vi "Texto Pasante.vi"() -> ()   [LabVIEW 2010]
panel:
  in  "Dejar espacio":bool
  in  "Columnas":u32=30
  out "Array booleano":bool[][](array[boolean])
  in  "Velocidad [columnas / segundo]":dbl(slide)=21.09090909090909 scale=1.0..40.0
  in  "Texto":string
  in  "Abrir fuente":bool
  in  "Salir":bool
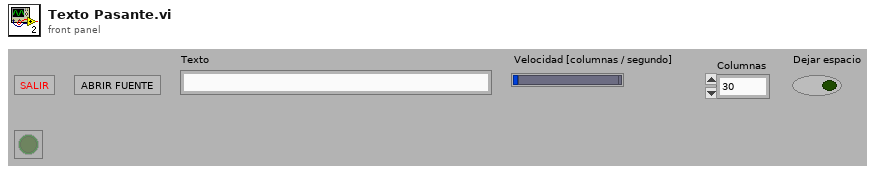
[diagram p1: front panel]
types:
  T1 = enum16{"open", "replace", "create", "open or create", "replace or create", "replace or create with confirmation"}
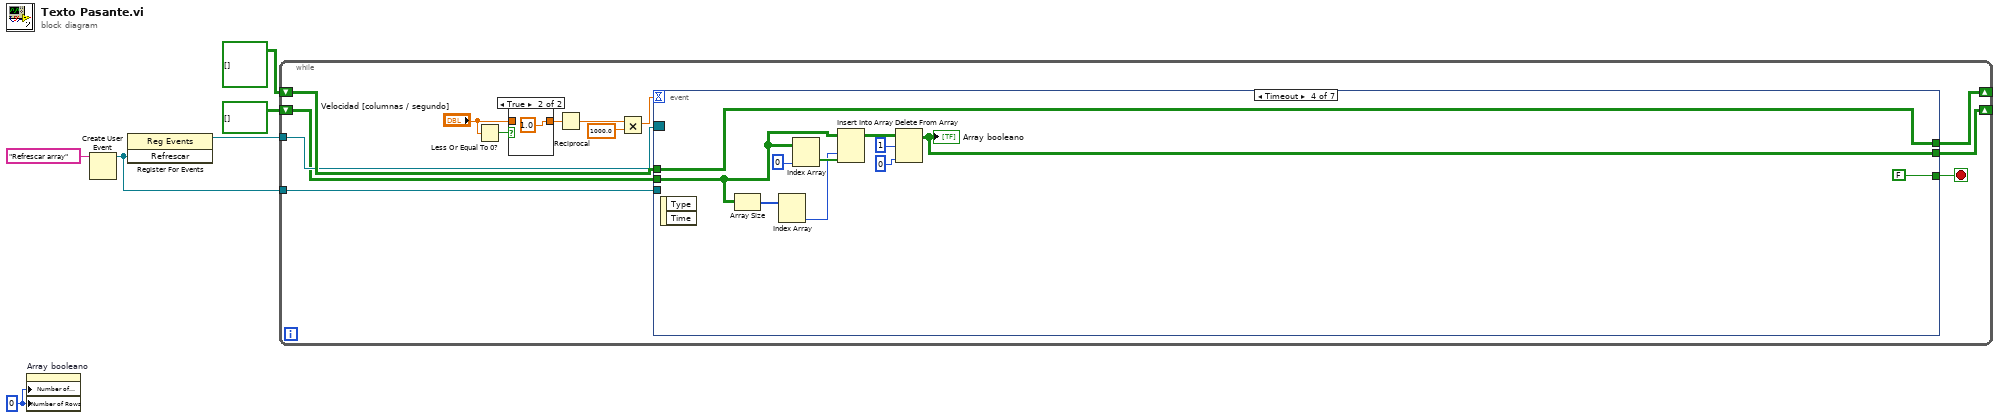
[diagram p0: block diagram]
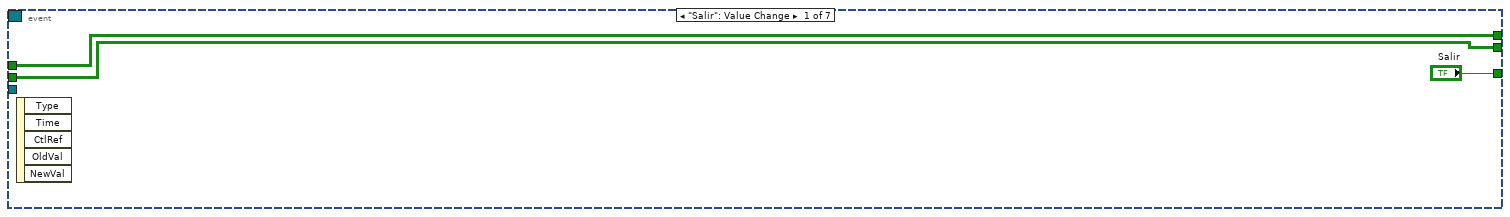
[diagram p3: hidden frame]
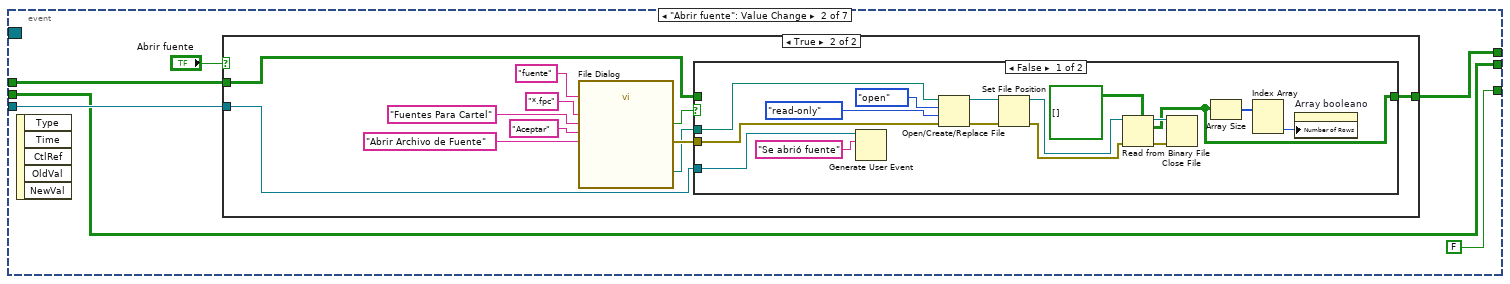
[diagram p4: hidden frame]
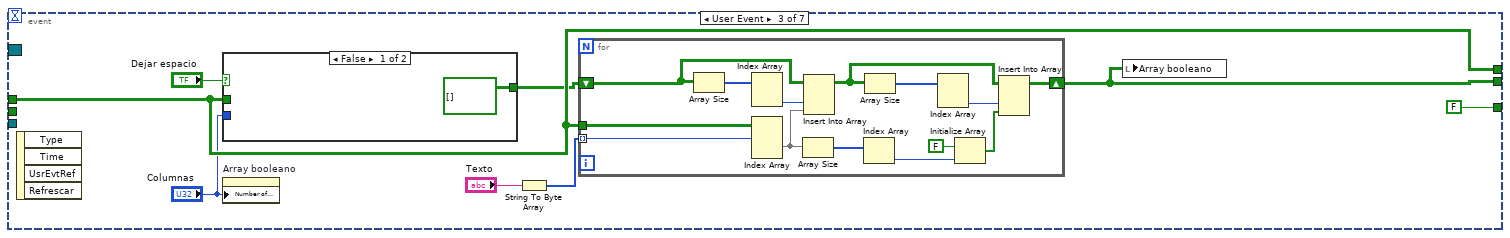
[diagram p7: hidden frame]
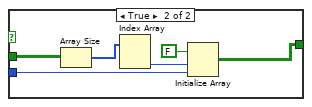
[diagram p8: hidden frame]
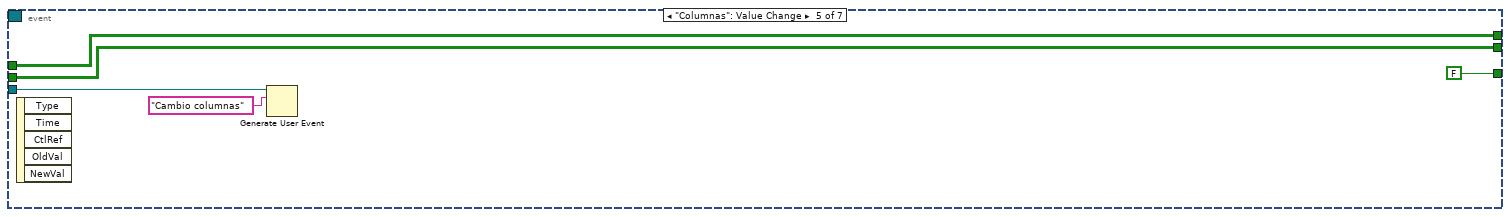
[diagram p9: hidden frame]
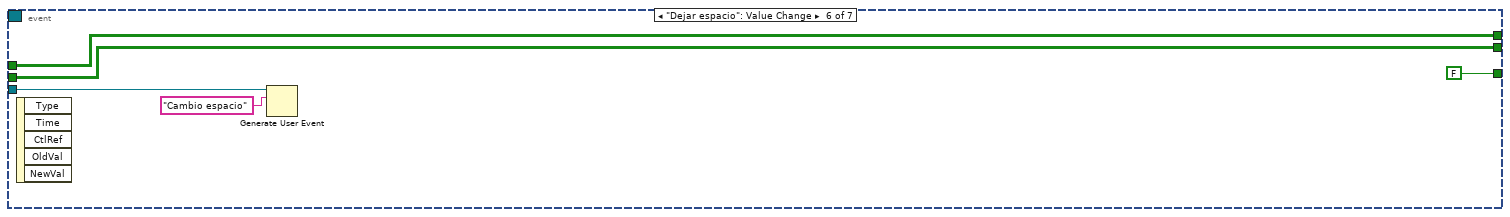
[diagram p10: hidden frame]
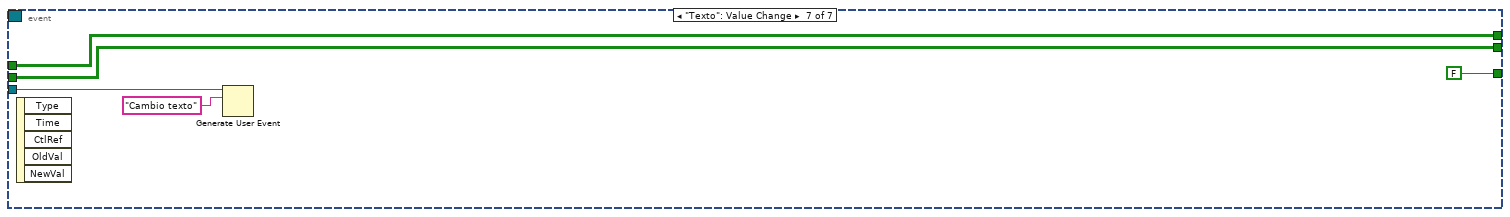
[diagram p11: hidden frame]
diagram:
  w1 = u32 0 ("Number of Columns")
  n1 = property on="Array booleano" class="Arr (strict)"("Number of Columns"=w1, "Number of Rows"=w1) -> ()  [unwired: 2 in, 2 out]
  n2 = Create User Event(user event datatype="Refrescar array" ("Refrescar")) -> (user event=w2:refnum<user-event>)  [unwired: 1 in, 1 out]
  n3 = register-events(w2) -> (reference out=w3:refnum<event-registration>)  [unwired: 2 in, 1 out]
  n4 = while {
    shift-right: [w17] -> _
    shift-left: bool[][][] [] ("appended array") -> [w18]
    shift-right: [w7] -> _
    shift-left: bool[][] [] ("Array booleano") -> [w14]
    tunnel: w3 -> [w16]
    tunnel: w2 -> [w15]
    stop <- w19 stop-if-true
    n5 = Less Or Equal To 0?(x="Velocidad [columnas / segundo]") -> (x <= 0?=w10:bool)
    n6 = case shown="True" w10 {
      tunnel: "Velocidad [columnas / segundo]" -> [w20 _]
      tunnel: [w20 1.0 ("Velocidad texto [caracteres/segundo]")] -> w11
      frame False {
      }
      frame True {
      }
    }
    n7 = Reciprocal(x=w11) -> (1/x=w12:dbl)
    n8 = Multiply(x=w12, y=1000.0) -> (x*y=w8:dbl)
    n9 = event shown="[3] Timeout" {
      selector: w16 -> [_ _ _ _ _ _ _]
      dyn-events: _ -> [_ _ _ _ _ _ _]
      timeout: w8 -> [_ _ _ _ _ _ _]
      tunnel: ["Salir" FALSE ("Salir") FALSE ("Salir") FALSE ("Salir") FALSE ("Salir") FALSE ("Salir") FALSE ("Salir")] -> w19
      tunnel: w18 -> [w23 w28 w62 w98 w103 w106 w111]
      tunnel: [w23 w27 w62 w98 w103 w106 w111] -> w17
      tunnel: w15 -> [_ w26 _ _ w102 w108 w113]
      tunnel: w14 -> [w22 w25 _ w96 w100 w107 w112]
      tunnel: [w22 w25 w64 w92 w100 w107 w112] -> w7
      event "Salir": Value Change {
        n10 = event-data() -> ()  [unwired: 1 in, 5 out]
      }
      event "Abrir fuente": Value Change {
        n11 = event-data() -> ()  [unwired: 1 in, 5 out]
        n12 = case shown="True" "Abrir fuente" {
          tunnel: [w31 w34] -> w27
          tunnel: w28 -> [w31 w33]
          tunnel: w26 -> [_ w32]
          frame False {
          }
          frame True {
            n13 = call "File Dialog"("prompt"="Abrir Archivo de Fuente", "button label"="Aceptar", "default name"="fuente", "pattern (all files)"="*.fpc", "pattern label"="Fuentes Para Cartel") -> ("selected path"=w35:path, "cancelled"=w37:bool, "error out"=w36:errorcluster)  [unwired: 7 in, 1 out]
            n14 = case shown="False" w37 {
              tunnel: w36 -> [w58 _]
              tunnel: w35 -> [w48 _]
              tunnel: [w47 w59] -> w34
              tunnel: w33 -> [_ w59]
              tunnel: w32 -> [w44 _]
              frame False {
                n15 = Generate User Event(user event=w44, event data cluster="Se abrió fuente" ("event data")) -> ()  [unwired: 1 in, 2 out]
                n16 = Open/Create/Replace File(file path (use dialog)=w48, error in=w58, operation (0:open)=T1."open", access (0:read/write)=enum16{"read/write", "read-only", "write-only"}."read-only") -> (refnum out=w54:refnum<file>, error out=w55:errorcluster)  [unwired: 2 in, 1 out]
                n17 = Set File Position(refnum=w54, error in=w55) -> (refnum out=w52:refnum<file>, error out=w53:errorcluster)  [unwired: 2 in]
                n18 = Read from Binary File(5:bool[][][] [] ("appended array"), 8:w53, 11:w52) -> (0:w50:errorcluster, 2:w47:bool[][][], 3:w51:refnum<file>)  [unwired: 3 in, 1 out]
                n19 = Close File(refnum=w51, error in=w50) -> ()  [unwired: 2 out]
                n20 = Array Size(array=w47) -> (size(s)=w46:i32[])
                n21 = Index Array(array=w46) -> (element #2=w45:i32)  [unwired: 2 in, 1 out]
                n22 = property on="Array booleano" class="Arr (strict)"("Number of Rows"=w45) -> ()  [unwired: 2 in, 2 out]
              }
              frame True {
              }
            }
          }
        }
      }
      event User Event {
        n23 = event-data() -> ()  [unwired: 1 in, 4 out]
        n24 = case shown="False" "Dejar espacio" {
          tunnel: w62 -> [_ w72]
          tunnel: "Columnas" -> [_ w70]
          tunnel: [bool[][] [] ("Array booleano") w69] -> w60
          frame False {
          }
          frame True {
            n25 = Array Size(array=w72) -> (size(s)=w74:i32[])
            n26 = Index Array(array=w74) -> (element #2=w71:i32)  [unwired: 2 in, 1 out]
            n27 = Initialize Array(FALSE, w71, w70) -> (w69:bool[][])
          }
        }
        n28 = property on="Array booleano" class="Arr (strict)"("Number of Columns"="Columnas") -> ()  [unwired: 2 in, 2 out]
        n29 = String To Byte Array(string="Texto") -> (unsigned byte array=w65:u8[])
        n30 = for {
          tunnel: w65 -> [w87] mode=indexing
          shift-right: [w82] -> w64
          shift-left: w60 -> [w86]
          tunnel: w62 -> [w88]
          n31 = Array Size(array=w86) -> (size(s)=w85:i32[])
          n32 = Index Array(array=w85) -> (element #2=w75:i32)  [unwired: 2 in, 1 out]
          n33 = Index Array(array=w88, index (dim 0)=w87) -> (element=w81:bool[][])  [unwired: 2 in]
          n34 = Array Size(array=w81) -> (size(s)=w80:i32[])
          n35 = Insert Into Array(array=w86, index (col)=w75, new element=w81) -> (w78:bool[][])  [unwired: 1 in]
          n36 = Index Array(array=w80) -> (element=w79:i32)  [unwired: 1 in]
          n37 = Array Size(array=w78) -> (size(s)=w77:i32[])
          n38 = Index Array(array=w77) -> (element #2=w76:i32)  [unwired: 2 in, 1 out]
          n39 = Initialize Array(FALSE, w79) -> (w83:bool[])
          n40 = Insert Into Array(array=w78, index (col)=w76, new element=w83) -> (w82:bool[][])  [unwired: 1 in]
        }
        n41 = local write "Array booleano"(w64) -> ()
      }
      event Timeout {
        n42 = event-data() -> ()  [unwired: 1 in, 2 out]
        n43 = Array Size(array=w96) -> (size(s)=w97:i32[])
        n44 = Index Array(array=w97) -> (element #2=w90:i32)  [unwired: 2 in, 1 out]
        n45 = Index Array(array=w96, index (col)=0 ("disabled index (col)")) -> (element=w95:bool[])  [unwired: 1 in]
        n46 = Insert Into Array(array=w96, index (col)=w90, new element=w95) -> (w94:bool[][])  [unwired: 1 in]
        n47 = Delete From Array(array=w94, length=1, index (col)=0 ("index (row)")) -> (array with subset deleted=w92:bool[][])  [unwired: 1 in, 1 out]
        "Array booleano" <- w92
      }
      event "Columnas": Value Change {
        n48 = event-data() -> ()  [unwired: 1 in, 5 out]
        n49 = Generate User Event(user event=w102, event data cluster="Cambio columnas" ("event data")) -> ()  [unwired: 1 in, 2 out]
      }
      event "Dejar espacio": Value Change {
        n50 = event-data() -> ()  [unwired: 1 in, 5 out]
        n51 = Generate User Event(user event=w108, event data cluster="Cambio espacio" ("event data")) -> ()  [unwired: 1 in, 2 out]
      }
      event "Texto": Value Change {
        n52 = event-data() -> ()  [unwired: 1 in, 5 out]
        n53 = Generate User Event(user event=w113, event data cluster="Cambio texto" ("event data")) -> ()  [unwired: 1 in, 2 out]
      }
    }
  }
